vi "Tree init parse.vi"(8 "error in (no error)":errorcluster, 11 "Tree ref":refnum<vi>) -> (0 "error out":errorcluster, 1 "map":T1[](array[typedef]), 2 "Selection Tags":string[](array[string]), 3 "Tree ref":refnum<vi>)   [LabVIEW 2020, in "UI_ItemSelect.lvlib"]
uses:
  UI_ItemSelect.lvlib
  Tree item selection indices.ctl
  tree item select search compare type.ctl
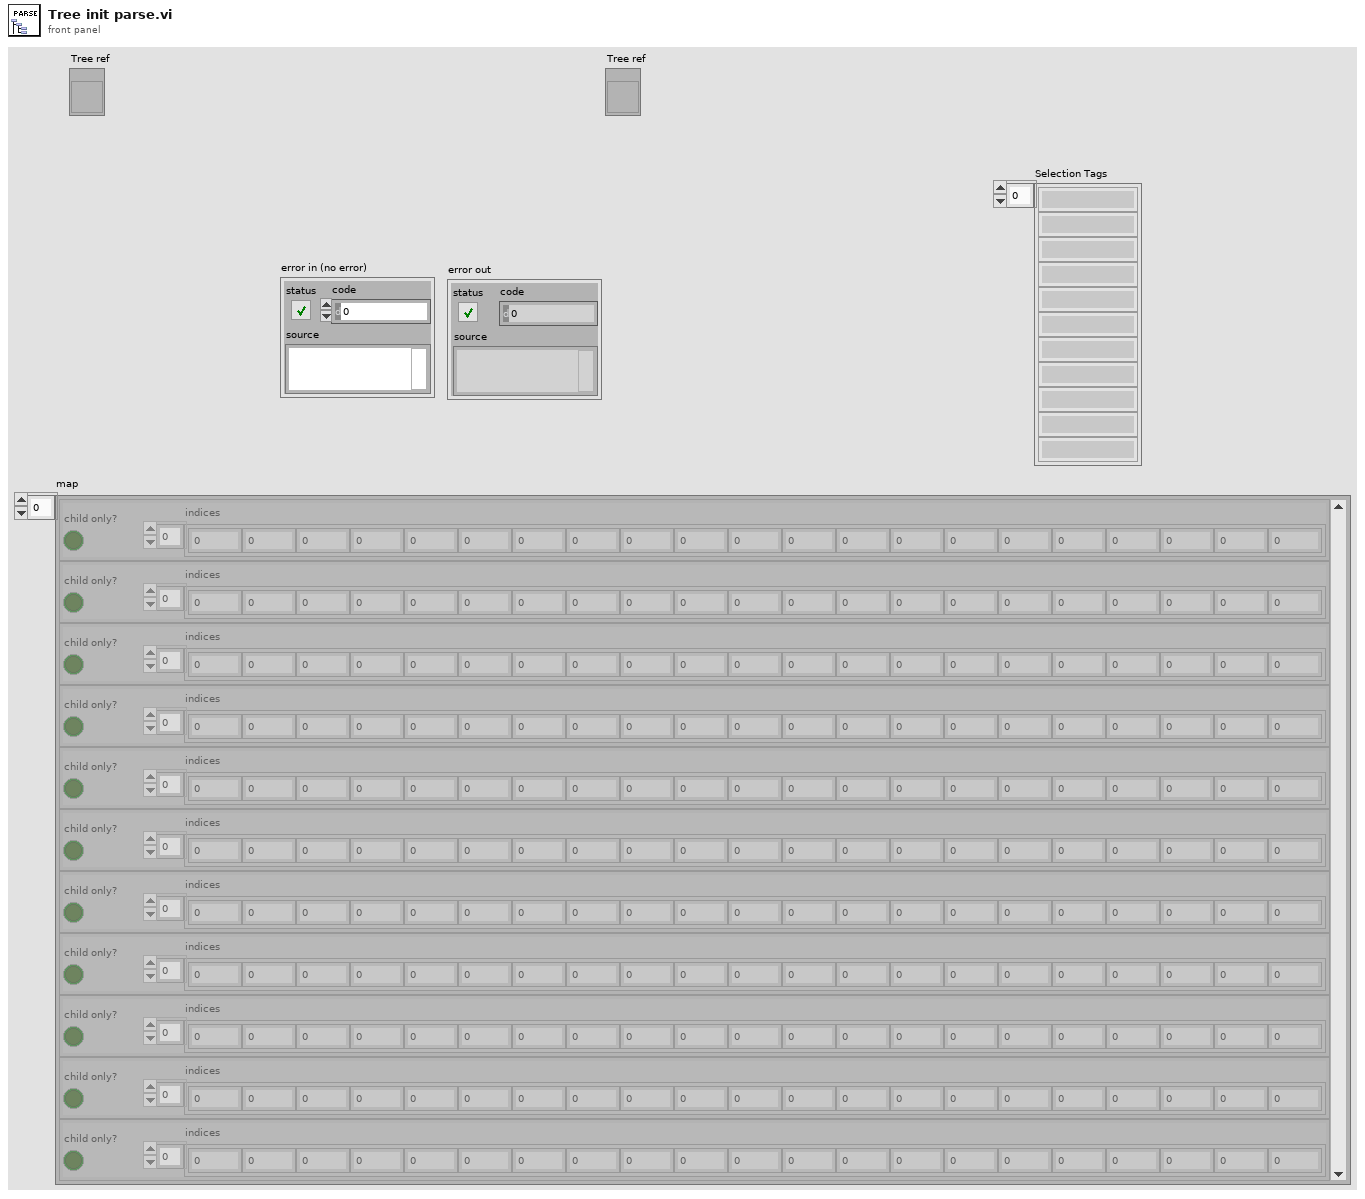
[diagram p1: front panel]
types:
  T1 = typedef "UI_ItemSelect.lvlib/Tree item selection indices.ctl" = cluster{"indices":i32[], "child only?":bool}
  T2 = typedef "UI_ItemSelect.lvlib/tree item select search compare type.ctl" = enum16{"less than", "less than or equal", "greater than", "greater than or equal"}
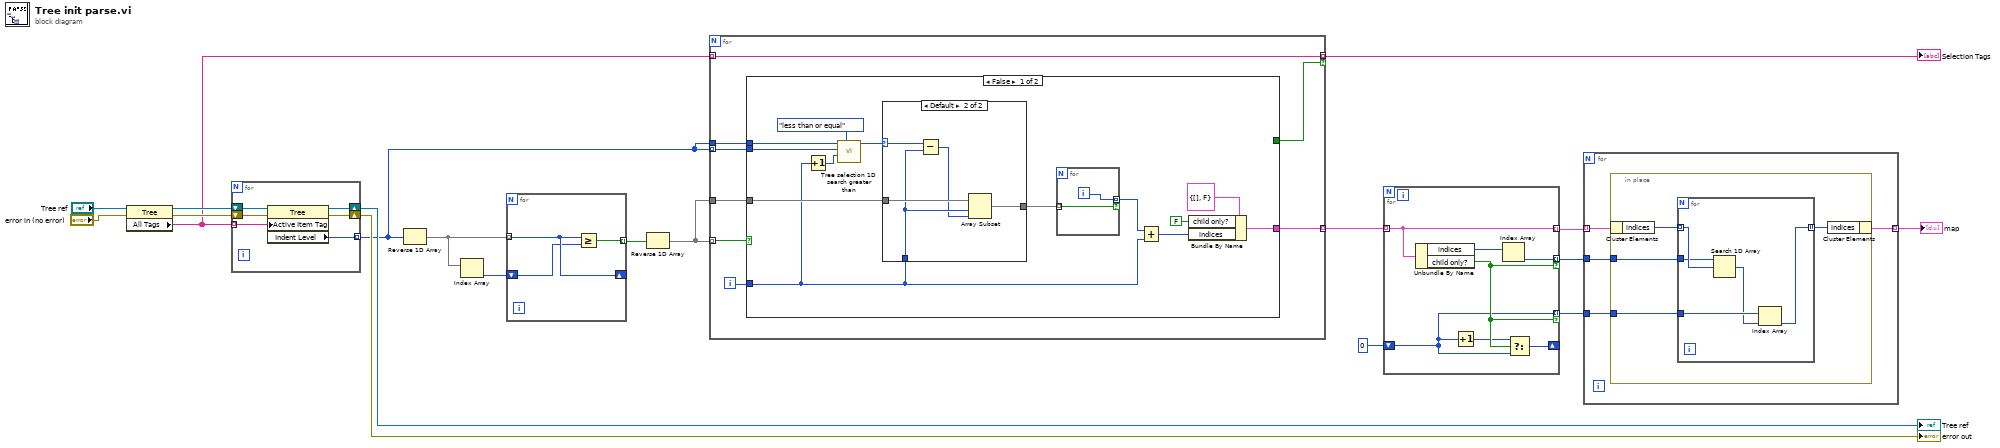
[diagram p0: block diagram]
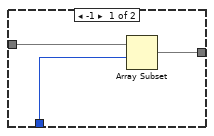
[diagram p2: hidden frame]
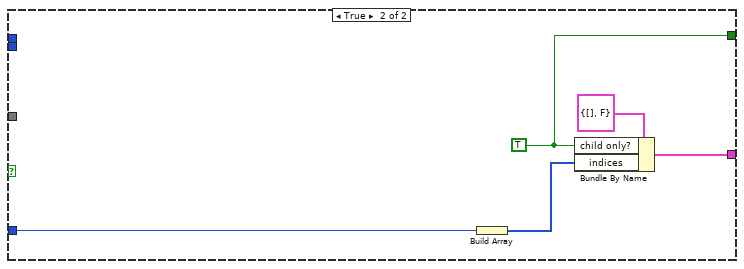
[diagram p3: hidden frame]
diagram:
  n1 = property class="Tree"(reference="Tree ref", error in="error in (no error)") -> (reference out=w19:refnum<vi>, error out=w15:errorcluster, "All Tags"=w4:string[])
  n2 = for {
    shift-right: [w23] -> w17
    shift-left: w19 -> [w25]
    tunnel: w4 -> [w24] mode=indexing
    tunnel: [w22] -> w3 mode=indexing
    shift-right: [w20] -> w14
    shift-left: w15 -> [w21]
    n3 = property class="Tree"(reference=w25, error in=w21, "Active Item Tag"=w24) -> (reference out=w23:refnum<vi>, error out=w20:errorcluster, "Indent Level"=w22:i32)
  }
  "Tree ref" <- w17
  "error out" <- w14
  n4 = Reverse 1D Array(array=w3) -> (reversed array=w13:i32[])
  n5 = Index Array(array=w13) -> (element=w12:i32)  [unwired: 1 in]
  n6 = for {
    tunnel: w13 -> [w28] mode=indexing
    shift-right: [w28] -> _
    shift-left: w12 -> [w27]
    tunnel: [w26] -> w11 mode=indexing
    n7 = Greater Or Equal?(x=w28, y=w27) -> (x >= y?=w26:bool)
  }
  n8 = Reverse 1D Array(array=w11) -> (reversed array=w10:bool[])
  n9 = for {
    tunnel: w3 -> [w36] mode=indexing
    tunnel: w10 -> [w34]
    tunnel: w3 -> [w35]
    tunnel: w10 -> [w32] mode=indexing
    tunnel: [w31] -> w2 mode=indexing
    tunnel: w4 -> [w30] mode=indexing
    tunnel: [w30] -> w5 mode=indexing if=w29
    i -> [w33]
    n10 = case shown="False" w32 {
      tunnel: w36 -> [w40 _]
      tunnel: w35 -> [w41 _]
      tunnel: w34 -> [w49 _]
      tunnel: w33 -> [w48 w64]
      tunnel: [w47 w62] -> w31
      tunnel: [_ w61] -> w29
      frame False {
        n11 = Increment(x=w48) -> (x+1=w39:i32)
        n12 = call "Tree selection 1D search greater than.vi"("Compare type"=tree_item_select_search_compare_type."less than or equal", "Start index (0)"=w39, "Element"=w40, "1D array"=w41) -> ("index of element"=w38:i32)  [unwired: 7 in]
        n13 = case shown="Default" w38 {
          selector: w38 -> [_ w56]
          tunnel: w49 -> [w52 w57]
          tunnel: w48 -> [w51 w55]
          tunnel: [w50 w53] -> w46
          frame -1 {
            n14 = Array Subset(array=w52, index=w51) -> (w50:bool[])  [unwired: 1 in]
          }
          frame Default {
            n15 = Subtract(x=w56, y=w55) -> (x-y=w54:i32)
            n16 = Array Subset(array=w57, index=w55, length=w54) -> (w53:bool[])
          }
        }
        n17 = for {
          tunnel: w46 -> [w58] mode=indexing
          tunnel: [w59] -> w45 mode=indexing if=w58
          i -> [w59]
        }
        n18 = Add(x=w45, y=w48) -> (x+y=w44:i32[])
        n19 = Bundle By Name(cluster=T1 {"indices"=[], "child only?"=FALSE} ("Cluster"), "child only?"=FALSE, "indices"=w44) -> (w47:T1)
      }
      frame True {
        w61 = TRUE ("child only?")
        n20 = Build Array(w64) -> (w63:i32[])
        n21 = Bundle By Name(cluster=T1 {"indices"=[], "child only?"=FALSE} ("Cluster"), "child only?"=w61, "indices"=w63) -> (w62:T1)
      }
    }
  }
  "Selection Tags" <- w5
  n22 = for {
    tunnel: w2 -> [w71] mode=indexing
    tunnel: [w65] -> w8 mode=indexing if=w68
    tunnel: [w71] -> w9 mode=indexing
    tunnel: [w69] -> w7 mode=indexing if=w68
    shift-right: [w66] -> _
    shift-left: 0 -> [w65]
    n23 = Unbundle By Name(w71) -> ("indices"=w70:i32[], "child only?"=w68:bool)
    n24 = Increment(x=w65) -> (x+1=w67:i32)
    n25 = Index Array(array=w70) -> (element=w69:i32)  [unwired: 1 in]
    n26 = Select(t=w67, s=w68, f=w65) -> (s? t:f=w66:i32)
  }
  n27 = for {
    tunnel: w9 -> [w75] mode=indexing
    tunnel: w8 -> [w73]
    tunnel: w7 -> [w74]
    tunnel: [w72] -> w1 mode=indexing
    n28 = in-place {
      in-place-border: w74 -> [w78]
      in-place-border: w73 -> [w77]
      n29 = in-place-cluster #1(w75) -> ("indices"=w79:i32[])
      n30 = for {
        tunnel: w79 -> [w84] mode=indexing
        tunnel: w78 -> [w83]
        tunnel: w77 -> [w82]
        tunnel: [w80] -> w76 mode=indexing
        n31 = Search 1D Array(1D array=w83, element=w84) -> (index of element=w81:i32)  [unwired: 1 in]
        n32 = Index Array(array=w82, index=w81) -> (element=w80:i32)
      }
      n33 = in-place-cluster #1("indices"=w76) -> (w72:T1)
    }
  }
  "map" <- w1
